vi "提取系统回应1.vi"(10 "字符串":string) -> (2 "系统回应":string, 3 "子字符串之前":string)   [LabVIEW 2014]
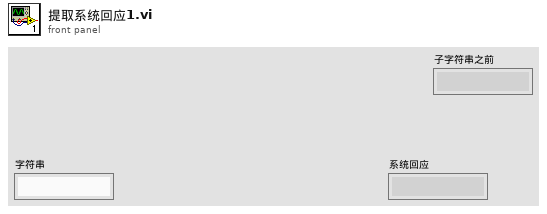
[diagram p1: front panel]
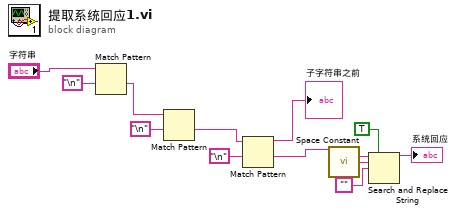
[diagram p0: block diagram]
diagram:
  n1 = Match Pattern(string="字符串", regular expression="\n") -> (after substring=w10:string)  [unwired: 1 in, 3 out]
  n2 = Match Pattern(string=w10, regular expression="\n") -> (after substring=w3:string)  [unwired: 1 in, 3 out]
  n3 = Match Pattern(string=w3, regular expression="\n") -> (before substring=→"子字符串之前":string, after substring=w2:string)  [unwired: 1 in, 2 out]
  n4 = call <vilib>:"Space Constant.vi"() -> ("String"=w9:string)
  n5 = Search and Replace String(replace all?=TRUE ("替换全部？(F)"), input string=w2, search string=w9, replace string="") -> (result string=→"系统回应":string)  [unwired: 4 in, 3 out]
